vi "Load_Max_Current.vi"(0 "Serial In":refnum<visa-resource-name>, 5 "Node":u8, 7 "Peak Current":bool, 9 "Max. Current":u16, 11 "Error In":errorcluster) -> (4 "Serial Out":refnum<visa-resource-name>, 15 "Error Out":errorcluster)   [LabVIEW 2019]
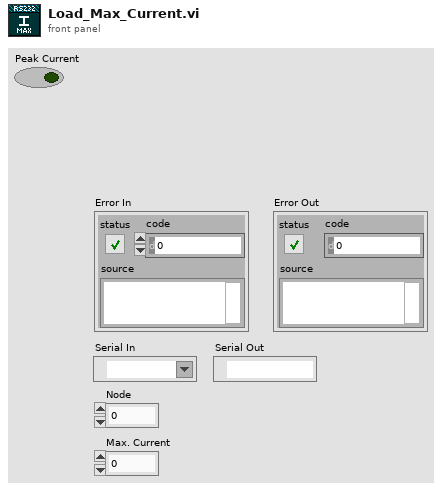
[diagram p1: front panel]
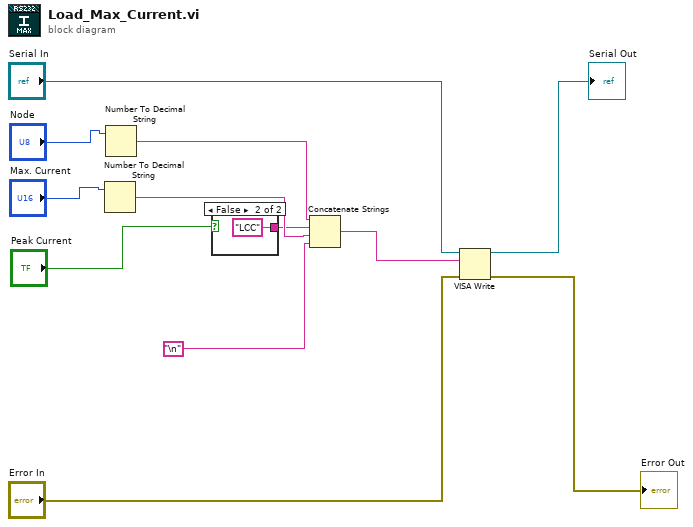
[diagram p0: block diagram]
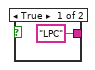
[diagram p2: hidden frame]
diagram:
  n1 = Number To Decimal String(number="Max. Current") -> (decimal integer string=w5:string)  [unwired: 1 in]
  n2 = Number To Decimal String(number="Node") -> (decimal integer string=w6:string)  [unwired: 1 in]
  n3 = case shown="False" "Peak Current" {
    tunnel: ["LPC" ("string") "LCC" ("string")] -> w3
    frame True {
    }
    frame False {
    }
  }
  n4 = Concatenate Strings(w6, w3, w5, "\n") -> (w4:string)
  n5 = VISA Write(VISA resource name="Serial In", write buffer=w4, error in (no error)="Error In") -> (VISA resource name out=→"Serial Out":refnum<visa-resource-name>, error out=→"Error Out":errorcluster)  [unwired: 1 out]
